vi "MW_Display_Python_Get_Frame.vi"(0 "session in":refnum<k35>, 5 "module path":path=path "D:/dev/Guy_Storage/Work/Cancun/MW_Display_Test/Magewell Capture/Capture_LV.py", 11 "error in":errorcluster, 12 "Frame Dims":T1) -> (4 "session out":refnum<k35>, 6 "module path out":path, 14 "RGB Pixels":u32[][](array[numeric]), 15 "error out":errorcluster)   [LabVIEW 2023]
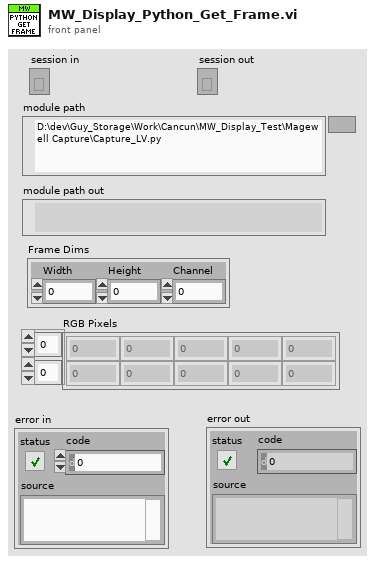
[diagram p1: front panel]
types:
  T1 = cluster{"Width":i32, "Height":i32, "Channel":i32}
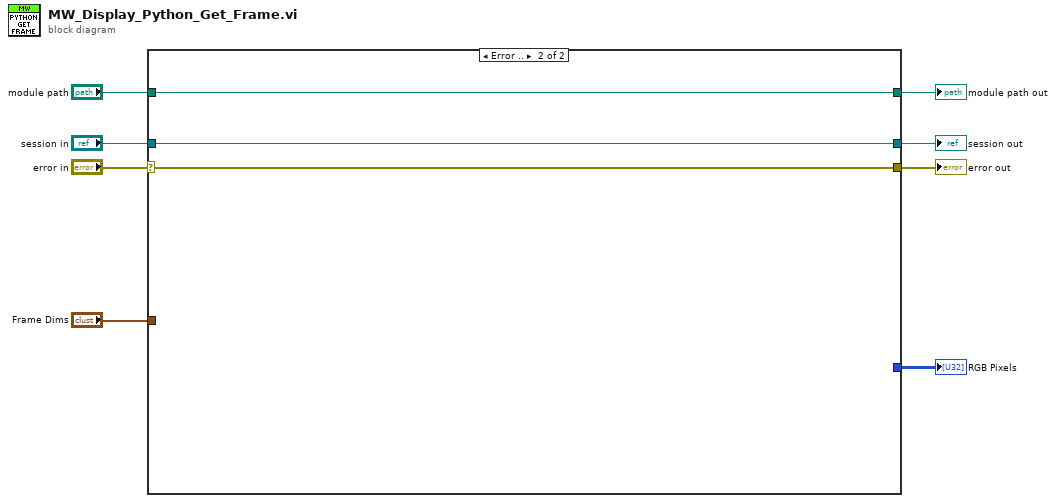
[diagram p0: block diagram]
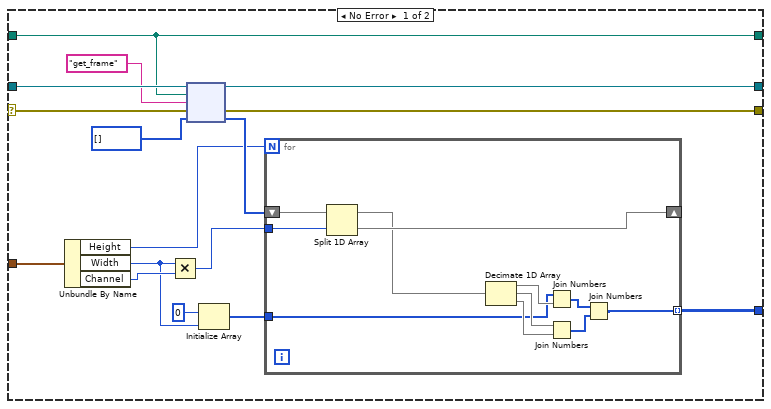
[diagram p2: hidden frame]
diagram:
  n1 = case shown="Error .." "error in" {
    selector: "error in" -> [w21 w37]
    tunnel: "module path" -> [w19 w36]
    tunnel: "session in" -> [w24 w38]
    tunnel: [w23 w37] -> w4
    tunnel: [w22 w38] -> w6
    tunnel: [w19 w36] -> w3
    tunnel: "Frame Dims" -> [w16 _]
    tunnel: [w9 _] -> w1
    frame No Error {
      n2 = Unbundle By Name(w16) -> ("Height"=w13:i32, "Width"=w11:i32, "Channel"=w15:i32)
      n3 = Multiply(x=w11, y=w15) -> (x*y=w14:i32)
      n4 = node(w24, w19, "get_frame" ("function name"), w21, u8[] []) -> (w22:refnum<k35>, w23:errorcluster, w17:u8[])  [unwired: 2 out]
      n5 = Initialize Array(u8 0, w11) -> (w10:u8[])
      n6 = for {
        N: w13 -> [_]
        tunnel: w14 -> [w34]
        shift-right: [w33] -> _
        shift-left: w17 -> [w35]
        tunnel: [w29] -> w9 mode=indexing
        tunnel: w10 -> [w25]
        n7 = Split 1D Array(array=w35, index=w34) -> (first subarray=w32:u8[], second subarray=w33:u8[])
        n8 = Decimate 1D Array(w32) -> (w26:u8[], w28:u8[], w27:u8[])
        n9 = Join Numbers(hi=w25, lo=w26) -> ((hi.lo)=w30:u16[])
        n10 = Join Numbers(hi=w28, lo=w27) -> ((hi.lo)=w31:u16[])
        n11 = Join Numbers(hi=w30, lo=w31) -> ((hi.lo)=w29:u32[])
      }
    }
    frame Error {
    }
  }
  "session out" <- w6
  "error out" <- w4
  "module path out" <- w3
  "RGB Pixels" <- w1
